vi "Sample Application.vi"(11 "Error in":errorcluster caption="Error in (no error)") -> (15 "Error out":errorcluster)   [LabVIEW 2018]
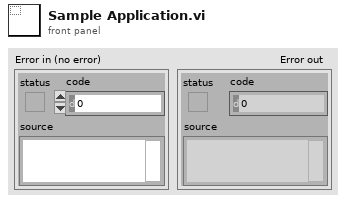
[diagram p1: front panel]
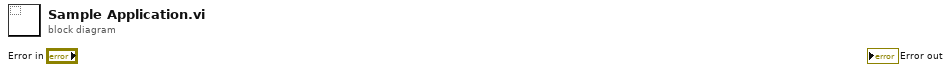
[diagram p0: block diagram]
diagram:
